vi "H-MEDI State Popup.vi"(8 "error in (no error)":errorcluster caption="에러 입력(에러 없음)") -> (0 "error out":errorcluster caption="에러 출력")   [LabVIEW 2019]
uses:
  03_Home/controller/pannelState.ctl
panel:
  in  "특이사항 및 개선할 것":string
  out "실험 결과":string
  out "메모":string
  in  "종료":bool
  in  "저장":bool
  # "실험 결과"
  # "메모"
  # "특이사항 및 개선할 것"
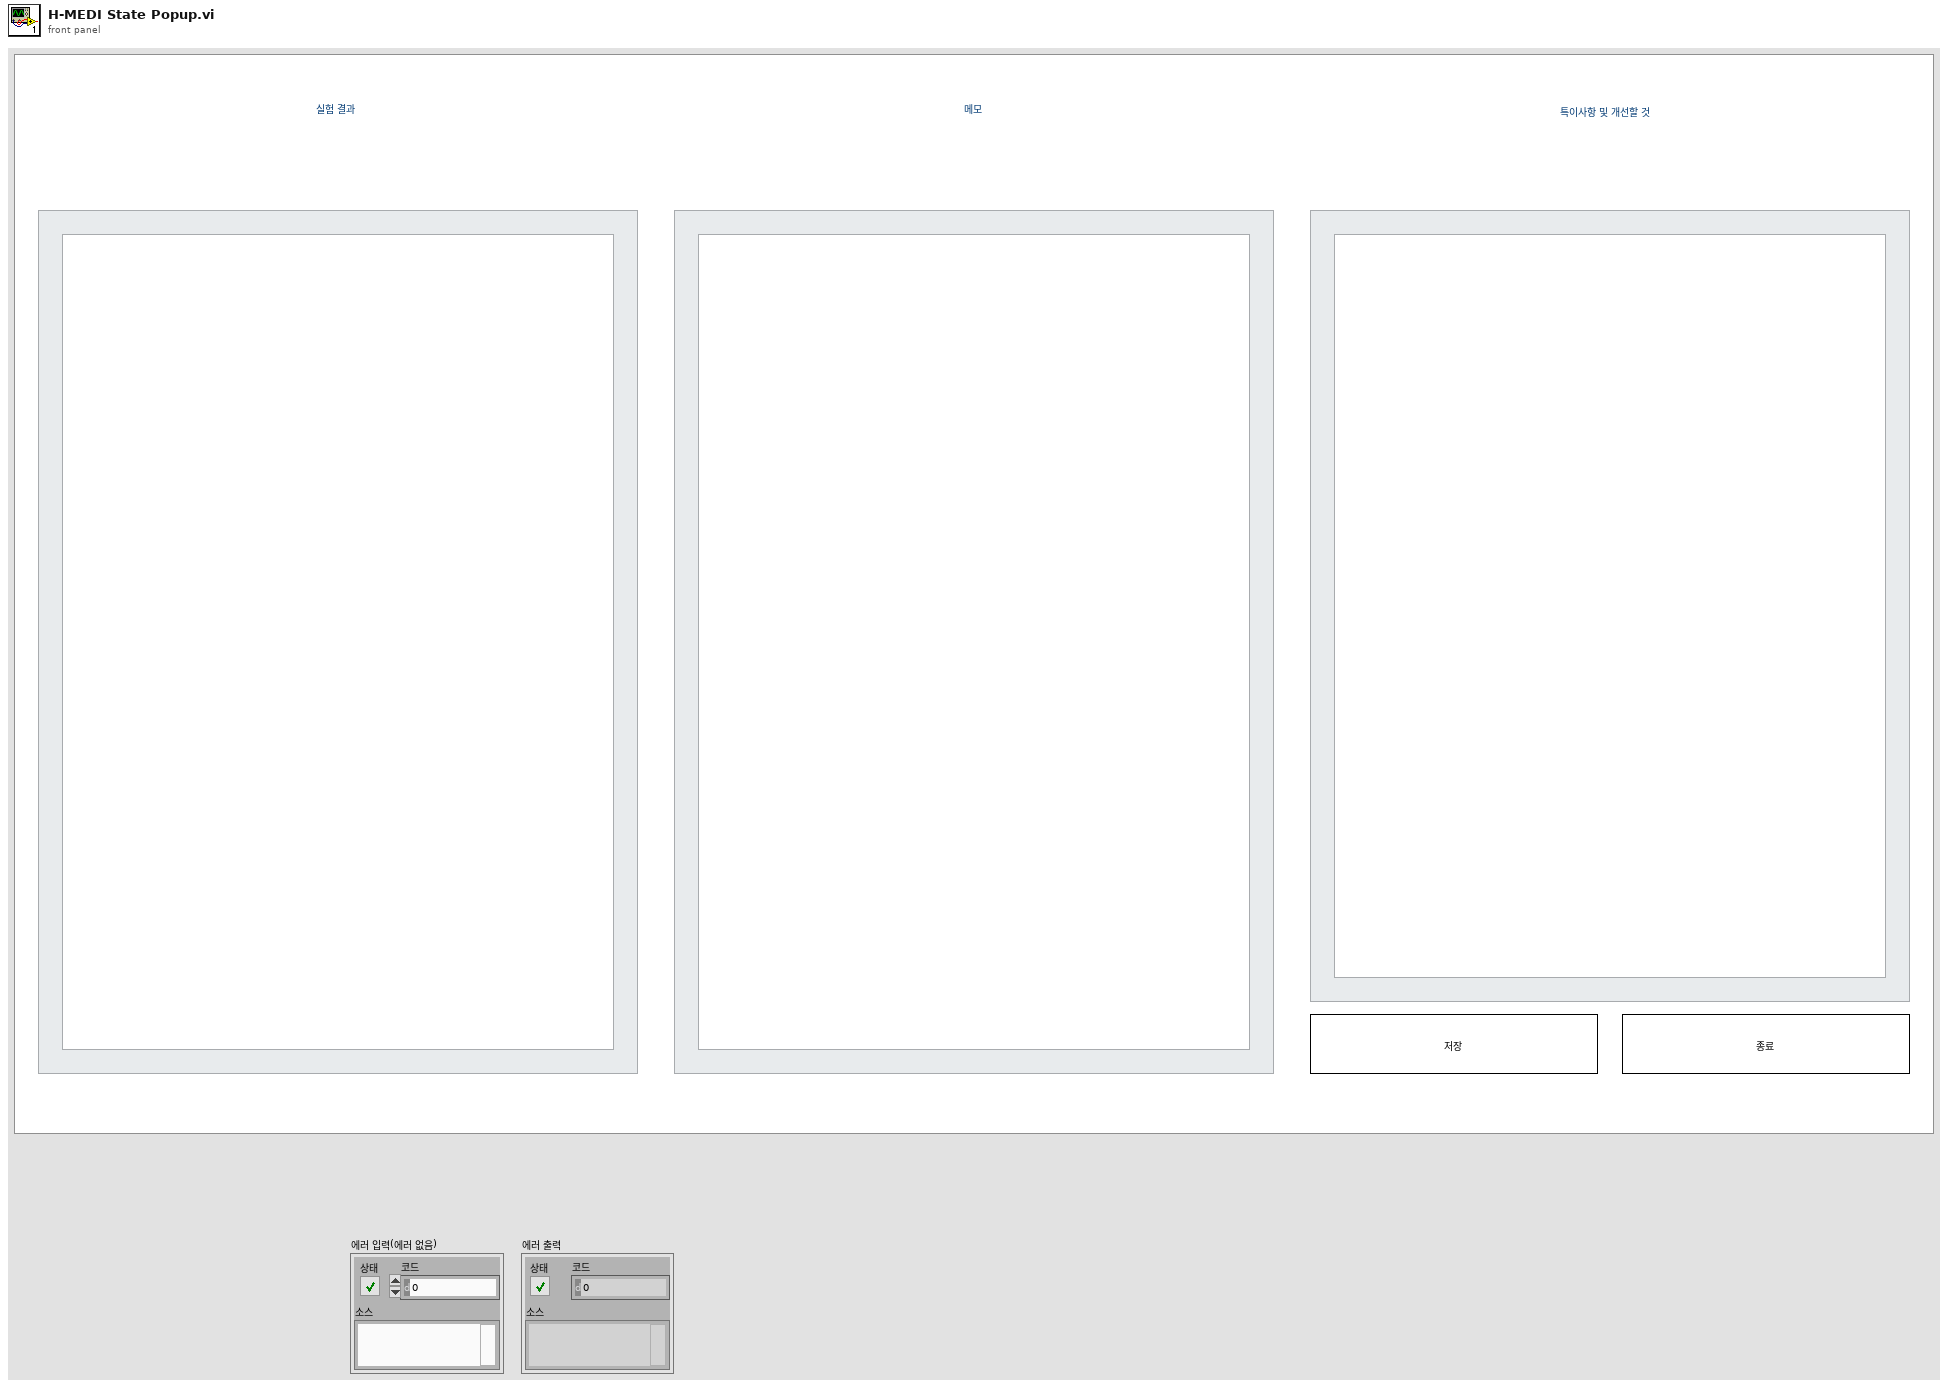
[diagram p1: front panel]
types:
  T1 = typedef "pannelState.ctl" = enum16{"Init", "LogIn", "SignUpView", "Home", "Management_patientList", "Management_patientTrashtList", "Management_patientCreate", "Management_patientUpdate", "Management_patientTraining", "Management_patientTrainingDetail", "H-MEDI PatientList", "H-MEDI HardwareCtl", "Adjust", "FineTuning", "UserList", "UserDetail", "Exit"}
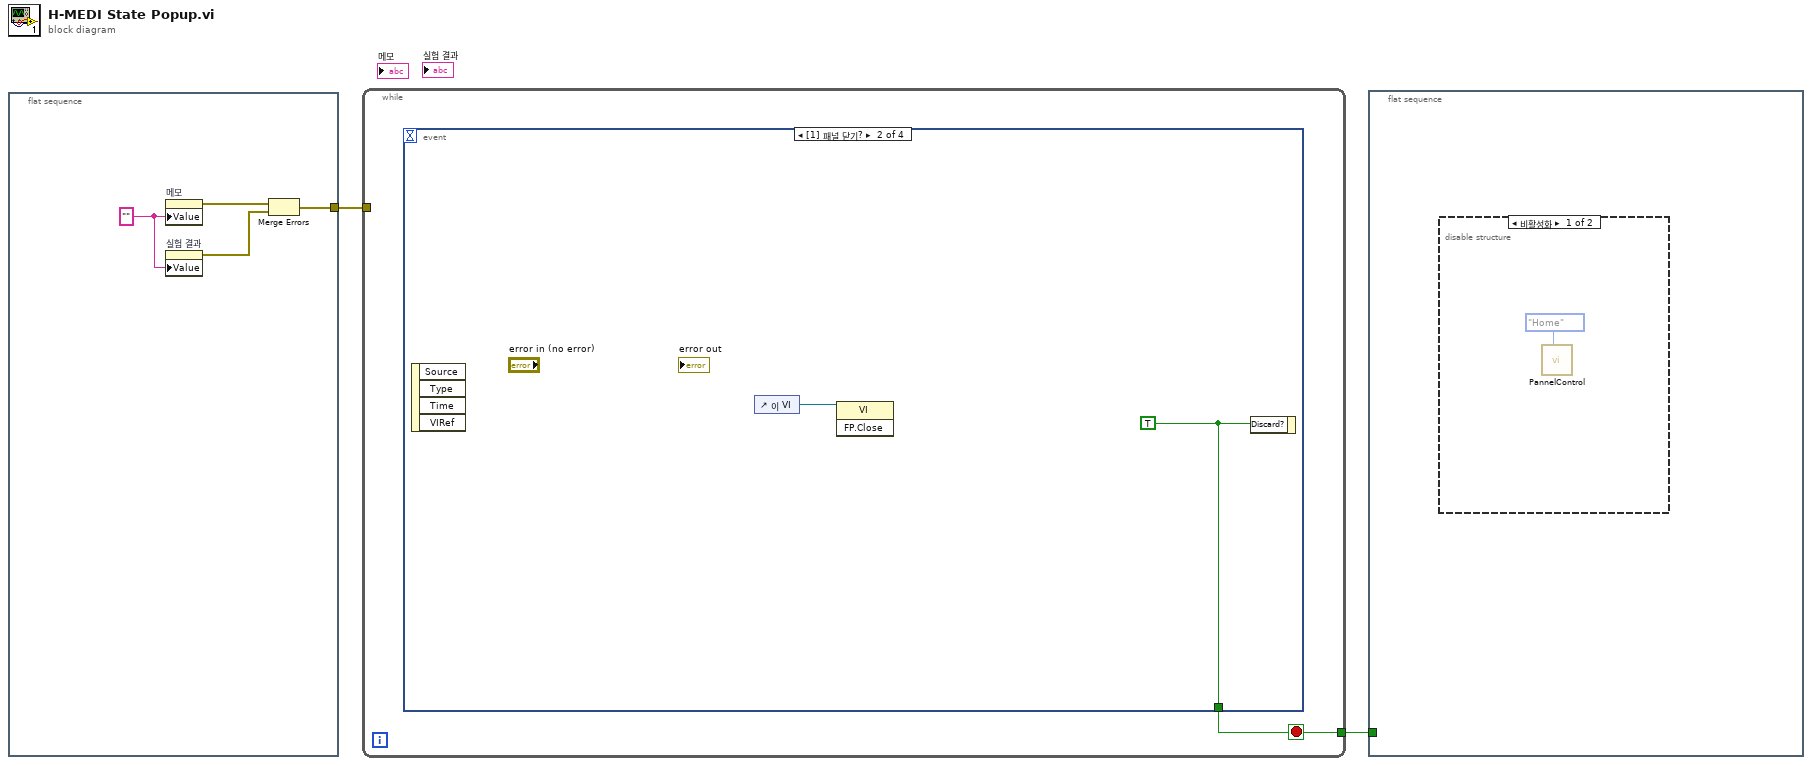
[diagram p0: block diagram]
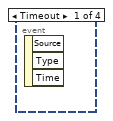
[diagram p3: hidden frame]
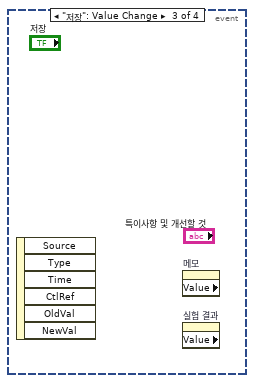
[diagram p4: hidden frame]
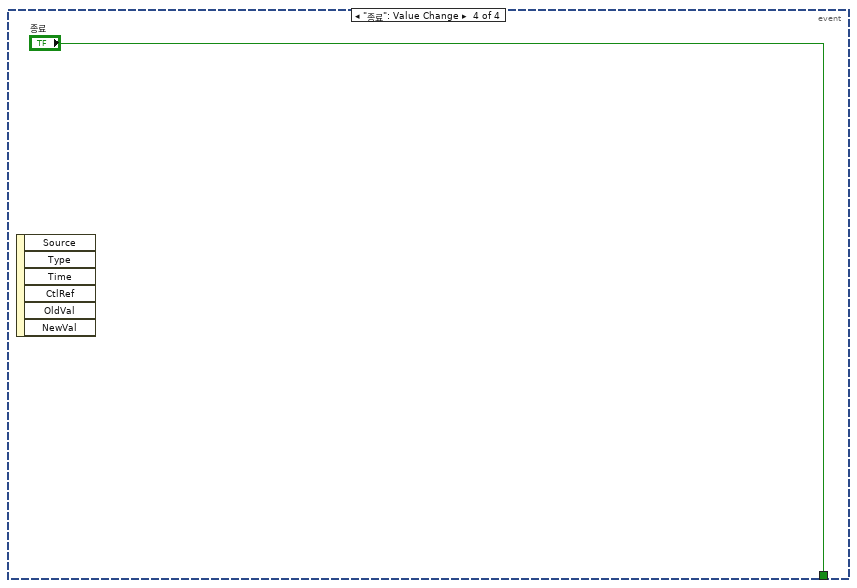
[diagram p5: hidden frame]
diagram:
  n1 = flat-sequence {
    tunnel: [w3] -> w2
    frame #0 {
      w6 = "" ("메모")
      n2 = property on="메모" class="Str"("Value"=w6) -> (error out=w5:errorcluster)  [unwired: 2 in, 1 out]
      n3 = property on="실험 결과" class="Str"("Value"=w6) -> (error out=w4:errorcluster)  [unwired: 2 in, 1 out]
      n4 = Merge Errors(w5, w4) -> (w3:errorcluster)
    }
  }
  n5 = while {
    tunnel: w2 -> [_]
    tunnel: [w7] -> w1
    stop <- w7 stop-if-true
    n6 = event shown="[1] 패널 닫기?" {
      selector: _ -> [_ _ _ _]
      dyn-events: _ -> [_ _ _ _]
      timeout: _ -> [_ _ _ _]
      tunnel: [_ w8 _ "종료"] -> w7
      event Timeout {
        n7 = event-data() -> ()  [unwired: 1 in, 3 out]
      }
      event Panel Close? {
        w8 = TRUE
        n8 = event-data() -> ()  [unwired: 1 in, 4 out]
        n9 = control-ref of="이 VI"() -> (w9:refnum<vi>)
        n10 = invoke class="VI" method="FP.Close"(reference=w9) -> ()  [unwired: 2 in, 3 out]
        n11 = event-data("Discard?"=w8) -> ()  [unwired: 1 in, 1 out]
      }
      event "저장": Value Change {
        n12 = event-data() -> ()  [unwired: 1 in, 6 out]
        n13 = property on="메모" class="Str" props=["Value"]() -> ()  [unwired: 2 in, 3 out]
        n14 = property on="실험 결과" class="Str" props=["Value"]() -> ()  [unwired: 2 in, 3 out]
      }
      event "종료": Value Change {
        n15 = event-data() -> ()  [unwired: 1 in, 6 out]
      }
    }
  }
  n16 = flat-sequence {
    tunnel: w1 -> [_]
    frame #0 {
      n17 = disable-structure shown="비활성화" {
        frame Disabled {
          n18 = call "PannelControl.vi"("State"=pannelState."Home") -> ()  [unwired: 10 in, 1 out]
        }
        frame Enabled {
        }
      }
    }
  }
